vi "Add Text to Element.vi"(8 "error in (no error)":errorcluster, 9 "Text":string, 10 "Parent Element":refnum<k20>, 11 "DOM document":refnum<k20>) -> (0 "error out":errorcluster, 2 "Text Node":refnum<k20>, 3 "DOM document out":refnum<k20>)   [LabVIEW 2013]
uses:
  <resource>/objmgr/DOMUserDefRef.rc
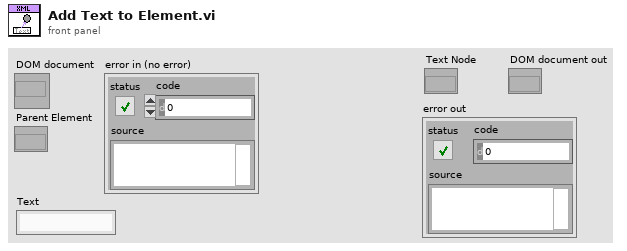
[diagram p1: front panel]
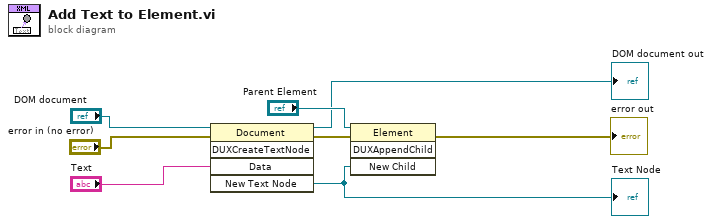
[diagram p0: block diagram]
diagram:
  n1 = invoke class="Document" method="DUXCreateTextNode"(reference="DOM document", error in="error in (no error)", "Data"="Text") -> (reference out=→"DOM document out":refnum<k20>, error out=w5:errorcluster, "New Text Node"=w3:refnum<k20>)  [unwired: 2 in, 2 out]
  "Text Node" <- w3
  n2 = invoke class="Element" method="DUXAppendChild"(reference="Parent Element", error in=w5, "New Child"=w3) -> (error out=→"error out":errorcluster)  [unwired: 1 in, 3 out]
